vi "Calculate_Linearity_Persentage_of_Subtrack-2.vi"(6 "[IN] Max angle":dbl, 7 "[IN] Subtrack":T1) -> (3 "[OUT] Track Linearity in %":u8)   [LabVIEW 2013]
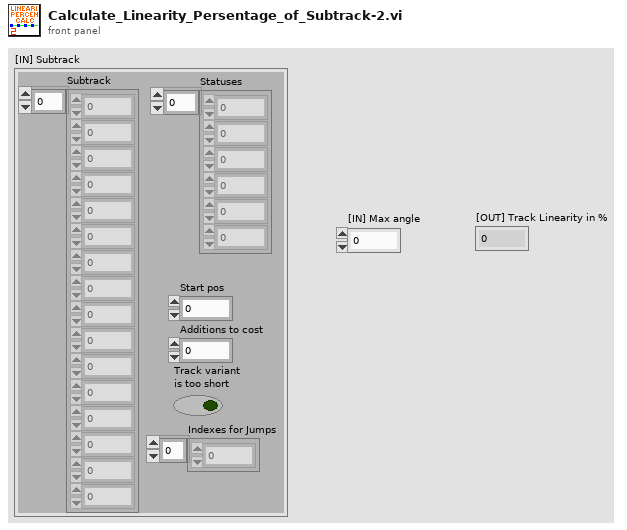
[diagram p1: front panel]
types:
  T1 = cluster{"Subtrack":dbl[], "Statuses":i16[], "Start pos":i32, "Additions to cost":i8, "Track variant \nis too short":bool, "Indexes for Jumps":i32[]}
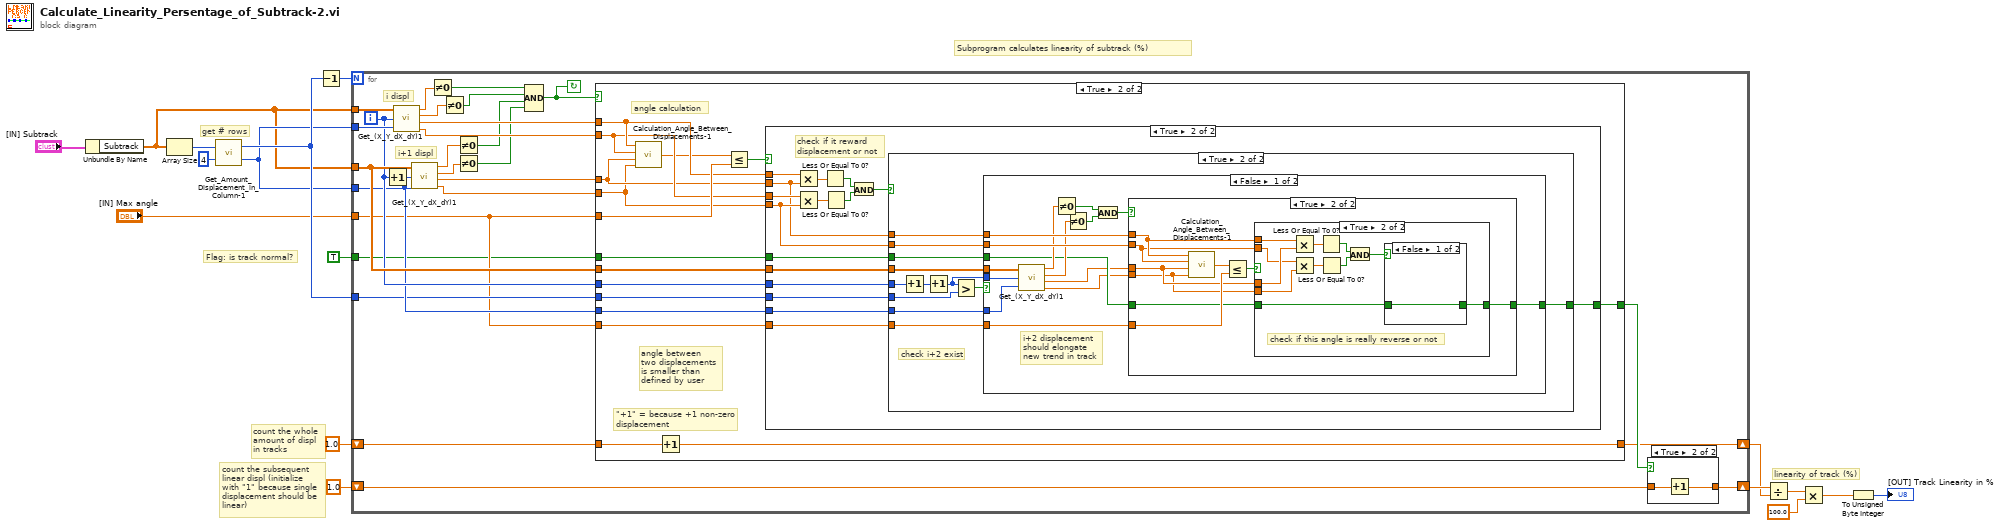
[diagram p0: block diagram]
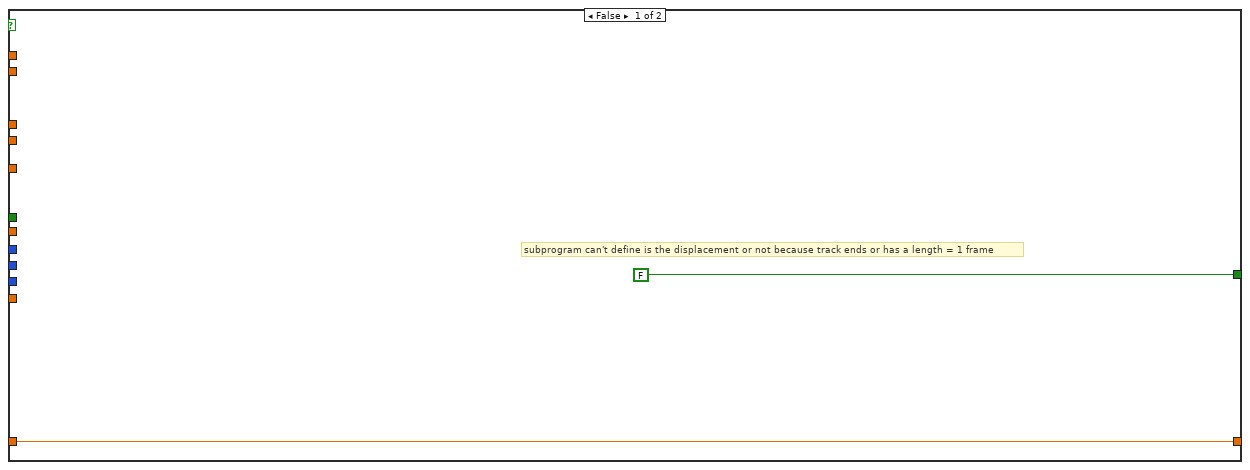
[diagram p3: hidden frame]
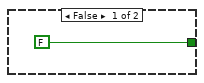
[diagram p4: hidden frame]
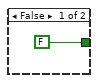
[diagram p6: hidden frame]
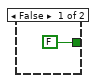
[diagram p7: hidden frame]
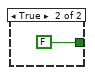
[diagram p8: hidden frame]
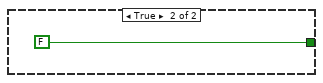
[diagram p9: hidden frame]
diagram:
  # "Subprogram calculates linearity of subtrack (%)"
  # "get # rows"
  # "linearity of track (%)"
  # "count the subsequent\nlinear displ (initialize \nwith \"1\" because single\ndisplacement should be\nlinear)"
  # "count the whole\namount of displ\nin tracks"
  # "Flag: is track normal?"
  n1 = Unbundle By Name("[IN] Subtrack") -> ("Subtrack"=w4:dbl[])
  n2 = Array Size(array=w4) -> (size(s)=w8:i32)
  n3 = call "Get_Amount_Displacement_in_Column-1.vi"("multiplier"=4, "# Rows"=w8) -> ("multiplier out"=w6:i32, "Displ amount"=w7:i32)
  n4 = Decrement(x=w7) -> (x-1=w17:i32)
  n5 = for {
    N: w17 -> [_]
    tunnel: w4 -> [w44]
    tunnel: w6 -> [w40]
    tunnel: w4 -> [w36]
    tunnel: w6 -> [w34]
    tunnel: "[IN] Max angle" -> [w29]
    tunnel: w7 -> [w30]
    tunnel: TRUE -> [w28]
    shift-right: [w25] -> w12
    shift-left: 1.0 -> [w26]
    shift-right: [w23] -> w13
    shift-left: 1.0 -> [w24]
    i -> [w35]
    stop <- w19 continue-if-true
    # "i+1 displ"
    # "i displ"
    n6 = Increment(x=w35) -> (x+1=w41:i32)
    n7 = call "Get_(X_Y_dX_dY)1.vi"("(X,Y,dX,dY)"=w44, "index"=w35, "multiplier"=w40) -> ("X"=w43:dbl, "Y"=w42:dbl, "dX"=w33:dbl, "dY"=w37:dbl)
    n8 = call "Get_(X_Y_dX_dY)1.vi"("(X,Y,dX,dY)"=w36, "index"=w41, "multiplier"=w34) -> ("X"=w39:dbl, "Y"=w38:dbl, "dX"=w32:dbl, "dY"=w31:dbl)
    n9 = Not Equal To 0?(x=w43) -> (x != 0?=w22:bool)
    n10 = Not Equal To 0?(x=w42) -> (x != 0?=w21:bool)
    n11 = Not Equal To 0?(x=w39) -> (x != 0?=w20:bool)
    n12 = Not Equal To 0?(x=w38) -> (x != 0?=w18:bool)
    n13 = Compound Arithmetic op=AND(w22, w21, w20, w18) -> (w19:bool)
    n14 = case shown="True" w19 {
      tunnel: w37 -> [_ w53]
      tunnel: w33 -> [_ w54]
      tunnel: w32 -> [_ w52]
      tunnel: w31 -> [_ w51]
      tunnel: w29 -> [_ w65]
      tunnel: w28 -> [_ w63]
      tunnel: [FALSE w62] -> w27
      tunnel: w36 -> [_ w61]
      tunnel: w35 -> [_ w60]
      tunnel: w34 -> [_ w59]
      tunnel: w30 -> [_ w58]
      tunnel: w29 -> [_ w57]
      tunnel: w26 -> [w49 w55]
      tunnel: [w49 w56] -> w25
      frame False {
        # "subprogram can't define is the displacement or not because track ends or has a length = 1 frame"
      }
      frame True {
        # "\"+1\" = because +1 non-zero\ndisplacement"
        # "angle calculation"
        # "angle between\ntwo displacements\nis smaller than \ndefined by user"
        n15 = call "Calculation_Angle_Between_Displacements-1.vi"("dY 2"=w51, "dX 2"=w52, "dY 1"=w53, "dX 1"=w54) -> ("angle in degrees"=w50:dbl)
        n16 = Increment(x=w55) -> (x+1=w56:dbl)
        n17 = Less Or Equal?(x=w50, y=w65) -> (x <= y?=w64:bool)
        n18 = case shown="True" w64 {
          tunnel: w52 -> [_ w67]
          tunnel: w51 -> [_ w69]
          tunnel: w54 -> [_ w82]
          tunnel: w53 -> [_ w70]
          tunnel: w63 -> [_ w76]
          tunnel: [FALSE w75] -> w62
          tunnel: w61 -> [_ w74]
          tunnel: w60 -> [_ w73]
          tunnel: w59 -> [_ w72]
          tunnel: w58 -> [_ w71]
          tunnel: w57 -> [_ w68]
          frame False {
          }
          frame True {
            # "check if it reward \ndisplacement or not"
            n19 = Multiply(x=w82, y=w67) -> (x*y=w81:dbl)
            n20 = Multiply(x=w70, y=w69) -> (x*y=w80:dbl)
            n21 = Less Or Equal To 0?(x=w81) -> (x <= 0?=w78:bool)
            n22 = Less Or Equal To 0?(x=w80) -> (x <= 0?=w79:bool)
            n23 = And(x=w78, y=w79) -> (x .and. y?=w77:bool)
            n24 = case shown="True" w77 {
              tunnel: w76 -> [w83 w91]
              tunnel: [w83 w90] -> w75
              tunnel: w74 -> [_ w89]
              tunnel: w73 -> [_ w95]
              tunnel: w72 -> [_ w87]
              tunnel: w71 -> [_ w93]
              tunnel: w67 -> [_ w86]
              tunnel: w69 -> [_ w85]
              tunnel: w68 -> [_ w84]
              frame False {
              }
              frame True {
                # "check i+2 exist"
                n25 = Increment(x=w95) -> (x+1=w94:i32)
                n26 = Increment(x=w94) -> (x+1=w88:i32)
                n27 = Greater?(x=w88, y=w93) -> (0:w92:bool)
                n28 = case shown="False" w92 {
                  tunnel: w91 -> [w100 _]
                  tunnel: [w96 FALSE] -> w90
                  tunnel: w89 -> [w107 _]
                  tunnel: w88 -> [w106 _]
                  tunnel: w87 -> [w105 _]
                  tunnel: w86 -> [w104 _]
                  tunnel: w85 -> [w103 _]
                  tunnel: w84 -> [w99 _]
                  frame False {
                    # "i+2 displacement \nshould elongate\nnew trend in track"
                    n29 = call "Get_(X_Y_dX_dY)1.vi"("(X,Y,dX,dY)"=w107, "index"=w106, "multiplier"=w105) -> ("X"=w102:dbl, "Y"=w101:dbl, "dX"=w98:dbl, "dY"=w97:dbl)
                    n30 = Not Equal To 0?(x=w102) -> (x != 0?=w110:bool)
                    n31 = Not Equal To 0?(x=w101) -> (x != 0?=w109:bool)
                    n32 = And(x=w110, y=w109) -> (x .and. y?=w108:bool)
                    n33 = case shown="True" w108 {
                      tunnel: [FALSE w117] -> w96
                      tunnel: w104 -> [_ w116]
                      tunnel: w103 -> [_ w115]
                      tunnel: w98 -> [_ w114]
                      tunnel: w97 -> [_ w113]
                      tunnel: w100 -> [_ w118]
                      tunnel: w99 -> [_ w120]
                      frame False {
                      }
                      frame True {
                        n34 = call "Calculation_Angle_Between_Displacements-1.vi"("dY 2"=w113, "dX 2"=w114, "dY 1"=w115, "dX 1"=w116) -> ("angle in degrees"=w112:dbl)
                        n35 = Less Or Equal?(x=w112, y=w120) -> (x <= y?=w119:bool)
                        n36 = case shown="True" w119 {
                          tunnel: w116 -> [_ w128]
                          tunnel: w114 -> [_ w127]
                          tunnel: w113 -> [_ w126]
                          tunnel: w115 -> [_ w125]
                          tunnel: w118 -> [_ w123]
                          tunnel: [FALSE w122] -> w117
                          frame False {
                          }
                          frame True {
                            # "check if this angle is really reverse or not"
                            n37 = Multiply(x=w128, y=w127) -> (x*y=w132:dbl)
                            n38 = Multiply(x=w125, y=w126) -> (x*y=w131:dbl)
                            n39 = Less Or Equal To 0?(x=w132) -> (x <= 0?=w129:bool)
                            n40 = Less Or Equal To 0?(x=w131) -> (x <= 0?=w130:bool)
                            n41 = And(x=w129, y=w130) -> (x .and. y?=w124:bool)
                            n42 = case shown="False" w124 {
                              tunnel: w123 -> [w133 _]
                              tunnel: [w133 FALSE] -> w122
                              frame False {
                              }
                              frame True {
                              }
                            }
                          }
                        }
                      }
                    }
                  }
                  frame True {
                  }
                }
              }
            }
          }
        }
      }
    }
    n43 = case shown="True" w27 {
      tunnel: w24 -> [w45 w47]
      tunnel: [w45 w46] -> w23
      frame False {
      }
      frame True {
        n44 = Increment(x=w47) -> (x+1=w46:dbl)
      }
    }
  }
  n45 = Divide(x=w13, y=w12) -> (x/y=w11:dbl)
  n46 = Multiply(x=w11, y=100.0) -> (x*y=w2:dbl)
  n47 = To Unsigned Byte Integer(number=w2) -> (unsigned 8bit integer=→"[OUT] Track Linearity in %":u8)
